vi "Shoot Comman.vi"(6 "Synchronization":enum16{"Start", "Wait"}(ring), 7 "Description":string, 8 "Command Info In":T3, 11 "Soft Shot?":bool) -> (0 "Command Info Out":T3)   [LabVIEW 2019]
doc: "This template has a parameter to control whether it waits for the command to complete or not. This is useful for operations that have a timed duration or a sensor-based duration. \n\nBe sure to right-click and select New from Template and save with a new command name."
uses:
  <vilib>/Rock Robotics/WPI/Framework/Command Status Info.ctl
  <vilib>/Rock Robotics/WPI/Framework/Completion Status.ctl
  <vilib>/Rock Robotics/WPI/Framework/Completion Notifier.ctl
  Implementation/Sequencer Type.ctl
  Implementation/All Commands.ctl
  Implementation/Subsystem Sequencer Setpoints.ctl
  Implementation/Subsystem Sequencer Operations.ctl
panel:
  in  "Soft":T1[](array[typedef])=[{"Cmd"=enum."Gripper - Gripper Shoot", "Value"=0.6}, {"Cmd"=enum."Wait ms", "Value"=800.0}, {"Cmd"=enum."Gripper - Gripper Stop", "Value"=0.0}]
  in  "Hard":T1[](array[typedef])=[{"Cmd"=enum."Gripper - Gripper Shoot", "Value"=1.0}, {"Cmd"=enum."Wait ms", "Value"=800.0}, {"Cmd"=enum."Gripper - Gripper Stop", "Value"=0.0}]
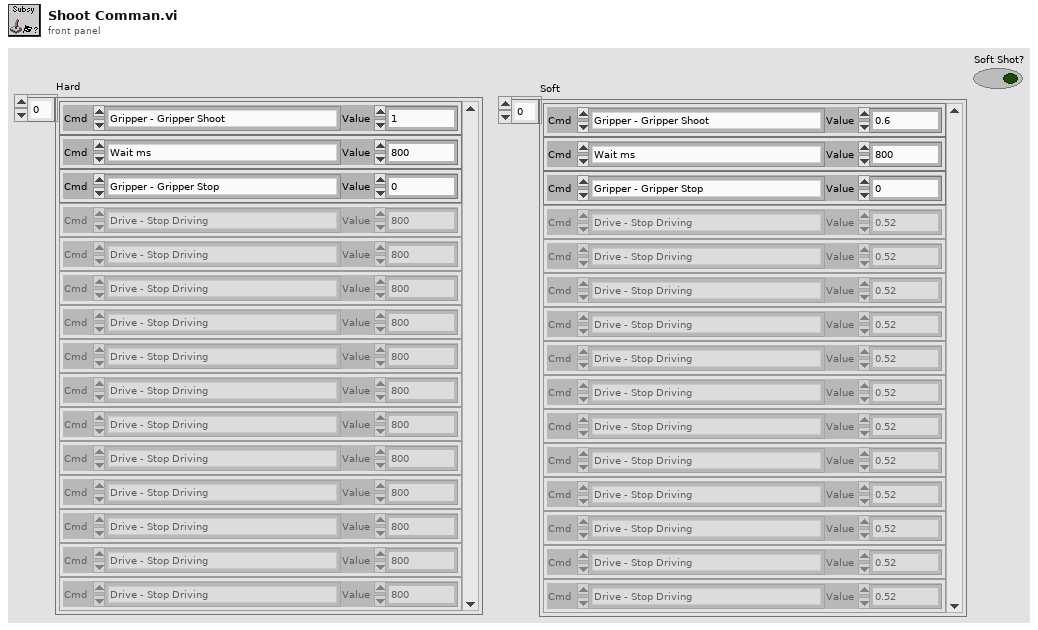
[diagram p1: front panel]
types:
  T1 = typedef "Sequencer Type.ctl" = cluster{"Cmd":T2, "Value":dbl}
  T2 = typedef "All Commands.ctl" = enum16{"Wait ms", "Drive - Stop Driving", "Drive - Set Shifter", "Drive - Drive Distance Straight", "Elevator - Elevator Stop", "Elevator - Elevator Set Position Wait", "Elevator - Elevator Set Position Start", "Arm - Arm to Shoot Position", "Arm - Arm to Pickup Position", "Arm - Arm Set Position", "Gripper - Gripper Stop", "Gripper - Gripper Shoot", "Gripper - Gripper Open", "Gripper - Gripper Intake", "Gripper - Gripper Close", "Gripper - Wait on Sensor"}
  T3 = typedef "Command Status Info.ctl" = cluster{"Name":string, "Status":T4, "notifier out":T5}
  T4 = typedef "Completion Status.ctl" = enum16{"Successful", "Aborted", "Incomplete"}
  T5 = typedef "Completion Notifier.ctl" = refnum<notifier>
  T6 = typedef "Subsystem Sequencer Setpoints.ctl" = cluster{"Operation":T7, "Setpoint":dbl, "Duration":dbl}
  T7 = typedef "Subsystem Sequencer Operations.ctl" = enum16{"Reserve", "Read Current", "Run Sequence"}
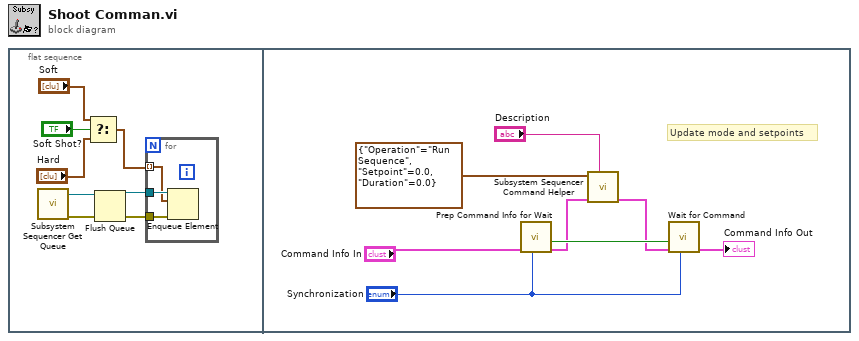
[diagram p0: block diagram]
diagram:
  n1 = flat-sequence {
    frame #0 {
      n2 = call "Subsystem Sequencer Get Queue.vi"() -> ("error out"=w6:errorcluster, "queue out"=w8:refnum<queue>)  [unwired: 10 in]
      n3 = Select(t="Soft", s="Soft Shot?", f="Hard") -> (s? t:f=w2:T1[])
      n4 = Flush Queue(queue=w8, error in (no error)=w6) -> (queue out=w7:refnum<queue>, error out=w5:errorcluster)  [unwired: 1 out]
      n5 = for {
        tunnel: w7 -> [w11]
        tunnel: w5 -> [w10]
        tunnel: w2 -> [w9] mode=indexing
        n6 = Enqueue Element(queue=w11, element=w9, error in (no error)=w10) -> ()  [unwired: 1 in, 3 out]
      }
    }
    frame #1 {
      # "Update mode and setpoints"
      n7 = call <vilib>:"Prep Command Info for Wait.vi"("Synchronication"="Synchronization", "Command Info"="Command Info In") -> ("Command Info"=w17:T3, "Allocated"=w18:bool)  [unwired: 8 in]
      n8 = call "Subsystem Sequencer Command Helper.vi"("Description"="Description", "Command Info In"=w17, "SubSystem Data"=T6 {"Operation"=enum."Run Sequence", "Setpoint"=0.0, "Duration"=0.0}) -> ("Command Info Out"=w14:T3)  [unwired: 6 in, 2 out]
      n9 = call <vilib>:"Wait for Command.vi"("Synchronication"="Synchronization", "Command Info in"=w14, "Allocated"=w18) -> ("Command Info out"=→"Command Info Out":T3)  [unwired: 8 in]
    }
  }
